vi "Serializer.Plaintext_Test.vi"() -> ()   [LabVIEW 2013]
uses:
  source/Serializer.PlainText/Serializer.PlainText.lvclass
panel:
  in  "Type Cast":bool
  out "error out":errorcluster
  out "Variant":variant
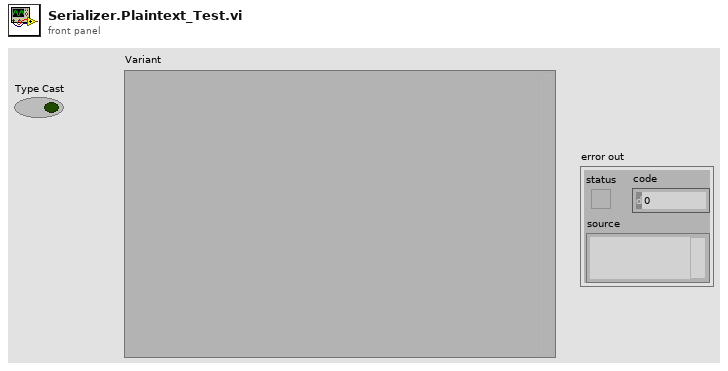
[diagram p1: front panel]
types:
  T1 = cluster{"Numeric":dbl, "Configuration Path":path, "Referenced?":bool, "Attribute":string}
  T2 = cluster{"Number1":dbl, "MyPath":path, "Initialized?":bool, "MyString with Spaces":string}
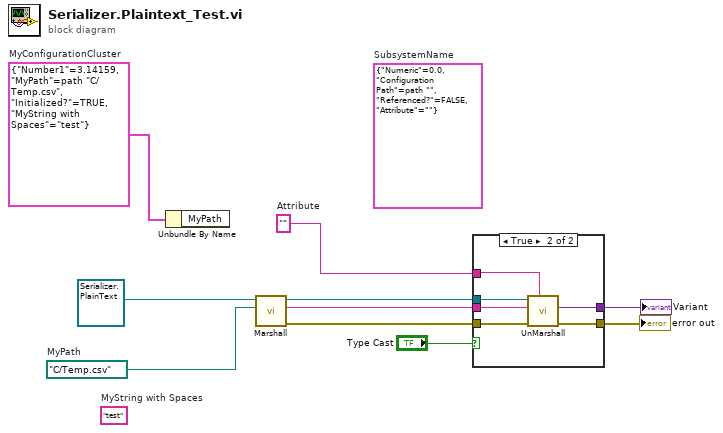
[diagram p0: block diagram]
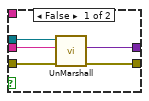
[diagram p2: hidden frame]
diagram:
  w1 = ""  # Attribute
  w2 = path "C:/Temp.csv"  # MyPath
  (unwired) "test"  # MyString with Spaces
  (unwired) T1 {"Numeric"=0.0, "Configuration Path"=path "", "Referenced?"=FALSE, "Attribute"=""}  # SubsystemName
  w3 = T2 {"Number1"=3.14159, "MyPath"=path "C:/Temp.csv", "Initialized?"=TRUE, "MyString with Spaces"="test"}  # MyConfigurationCluster
  n1 = Unbundle By Name(w3) -> ()  [unwired: 1 out]
  n2 = call-dynamic "Marshall.vi"("Variant"=w2, "Serializer in"=refnum<class "Serializer.PlainText.lvclass"> refnum ("CfgManager.Text.lvlib:Serializer.PlainText.lvclass")) -> ("error out"=w7:errorcluster, "String"=w9:string, "Serializer out"=w10:refnum<class "Serializer.PlainText.lvclass">)  [unwired: 7 in]
  n3 = case shown="True" "Type Cast" {
    tunnel: w10 -> [w15 w21]
    tunnel: w9 -> [w13 w20]
    tunnel: [w11 w19] -> w8
    tunnel: w7 -> [w14 w18]
    tunnel: [w12 w17] -> w6
    tunnel: w1 -> [_ w16]
    frame False {
      n4 = call-dynamic "UnMarshall.vi"("error in (no error)"=w14, "String"=w13, "Serializer in"=w15) -> ("error out"=w12:errorcluster, "Variant"=w11:variant)  [unwired: 6 in, 1 out]
    }
    frame True {
      n5 = call-dynamic "UnMarshall.vi"("Type"=w16, "error in (no error)"=w18, "String"=w20, "Serializer in"=w21) -> ("error out"=w17:errorcluster, "Variant"=w19:variant)  [unwired: 5 in, 1 out]
    }
  }
  "Variant" <- w8
  "error out" <- w6
